vi "byte0-19(SubVI).vi"(0 "unsigned byte array":u8[](array[numeric])) -> (1 "Numeric 2":u16, 2 "Numeric":u16, 3 "Numeric 9":u16, 4 "Numeric 10":u16, 6 "Numeric 3":u16, 8 "Numeric 8":u16, 10 "Numeric 7":u16, 12 "Numeric 4":u16, 13 "Numeric 5":u16, 14 "Numeric 6":u16)   [LabVIEW 2016]
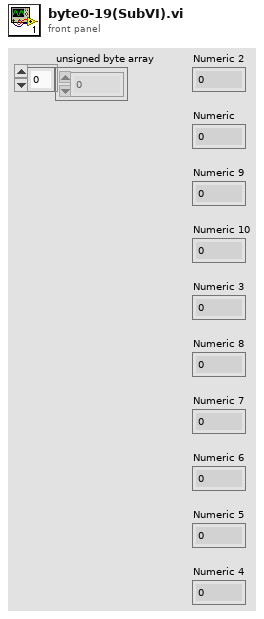
[diagram p1: front panel]
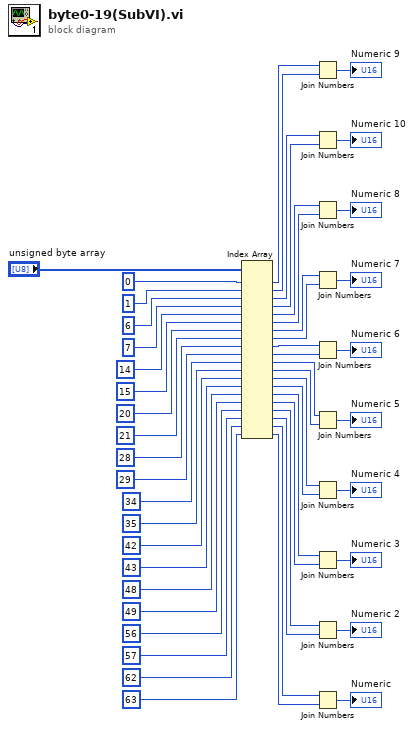
[diagram p0: block diagram]
diagram:
  n1 = Index Array(array="unsigned byte array", index #1=0 ("index"), index #2=1 ("index"), index #3=6 ("index"), index #4=7 ("index"), index #5=14 ("index"), index #6=15 ("index"), index #7=20 ("index"), index #8=21 ("index"), index #9=28 ("index"), index #10=29 ("index"), index #11=34 ("index"), index #12=35 ("index"), index #13=42 ("index"), index #14=43 ("index"), index #15=48 ("index"), index #16=49 ("index"), index #17=56 ("index"), index #18=57 ("index"), index #19=62 ("index"), index #20=63 ("index")) -> (element #1=w3:u8, element #2=w4:u8, element #3=w7:u8, element #4=w8:u8, element #5=w11:u8, element #6=w12:u8, element #7=w15:u8, element #8=w16:u8, element #9=w19:u8, element #10=w20:u8, element #11=w23:u8, element #12=w24:u8, element #13=w27:u8, element #14=w28:u8, element #15=w31:u8, element #16=w32:u8, element #17=w35:u8, element #18=w36:u8, element #19=w39:u8, element #20=w40:u8)
  n2 = Join Numbers(hi=w3, lo=w4) -> ((hi.lo)=→"Numeric 9":u16)
  n3 = Join Numbers(hi=w7, lo=w8) -> ((hi.lo)=→"Numeric 10":u16)
  n4 = Join Numbers(hi=w11, lo=w12) -> ((hi.lo)=→"Numeric 8":u16)
  n5 = Join Numbers(hi=w15, lo=w16) -> ((hi.lo)=→"Numeric 7":u16)
  n6 = Join Numbers(hi=w19, lo=w20) -> ((hi.lo)=→"Numeric 6":u16)
  n7 = Join Numbers(hi=w23, lo=w24) -> ((hi.lo)=→"Numeric 5":u16)
  n8 = Join Numbers(hi=w27, lo=w28) -> ((hi.lo)=→"Numeric 4":u16)
  n9 = Join Numbers(hi=w31, lo=w32) -> ((hi.lo)=→"Numeric 3":u16)
  n10 = Join Numbers(hi=w35, lo=w36) -> ((hi.lo)=→"Numeric 2":u16)
  n11 = Join Numbers(hi=w39, lo=w40) -> ((hi.lo)=→"Numeric":u16)
